vi "AssertError.vi"(8 "error in (no error)":errorcluster, 11 "Expected Error":T1=402902 items=["[5120] Invalid ID"=402902, "[5110] Failed to Init"=402900, "[5111] Unknown Error"=402901, "[5130] Save - Bad File Extension"=402903, "[5131] Save - General Error"=402904, "[5140] Unsupported (Polar)"=402905, "[5141] Unsupported (Logscale)"=402906, "[5142] Coordinates Not Regular"=402907]) -> (0 "error out":errorcluster)   [LabVIEW 2013]
uses:
  ErrorCodes.ctl
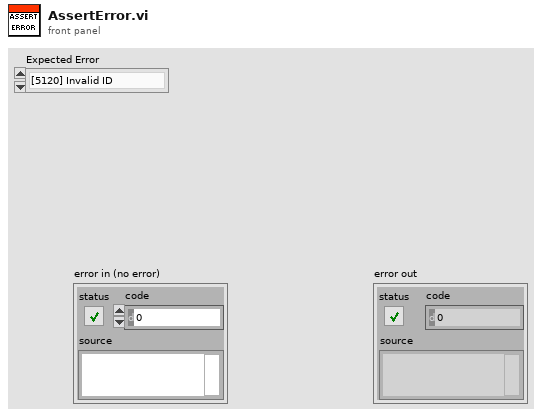
[diagram p1: front panel]
types:
  T1 = typedef "ErrorCodes.ctl" = u32
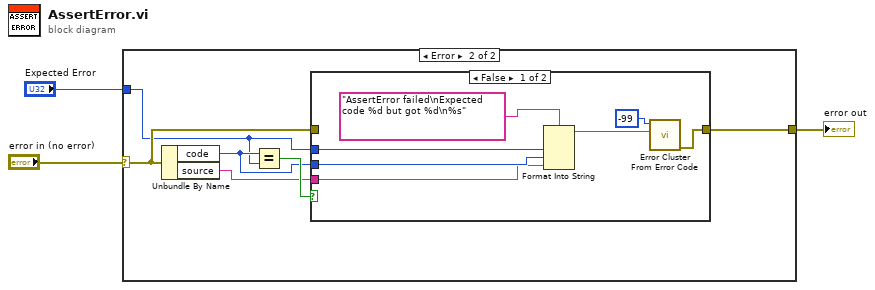
[diagram p0: block diagram]
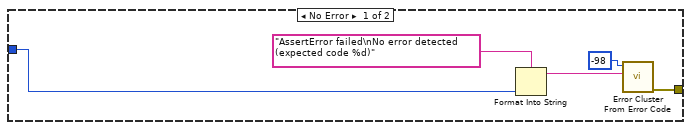
[diagram p2: hidden frame]
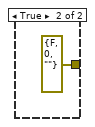
[diagram p3: hidden frame]
diagram:
  n1 = case shown="Error" "error in (no error)" {
    selector: "error in (no error)" -> [_ w13]
    tunnel: [w4 w12] -> w2
    tunnel: "Expected Error" -> [w7 w9]
    frame No Error {
      n2 = Format Into String(format string="AssertError failed\nNo error detected (expected code %d)", w7) -> (resulting string=w6:string)  [unwired: 2 in, 1 out]
      n3 = call <vilib>:"Error Cluster From Error Code.vi"("error message (\"\")"=w6, "error code (0)"=-98) -> ("error out"=w4:errorcluster)  [unwired: 7 in]
    }
    frame Error {
      n4 = Unbundle By Name(w13) -> ("code"=w11:i32, "source"=w10:string)
      n5 = Equal?(x=w11, y=w9) -> (x = y?=w14:bool)
      n6 = case shown="False" w14 {
        tunnel: w13 -> [_ _]
        tunnel: [w15 errorcluster {"status"=FALSE, "code"=0, "source"=""} ("error out")] -> w12
        tunnel: w9 -> [w20 _]
        tunnel: w11 -> [w19 _]
        tunnel: w10 -> [w18 _]
        frame False {
          n7 = Format Into String(format string="AssertError failed\nExpected code %d but got %d\n%s", w20, w19, w18) -> (resulting string=w16:string)  [unwired: 2 in, 1 out]
          n8 = call <vilib>:"Error Cluster From Error Code.vi"("error message (\"\")"=w16, "error code (0)"=-99) -> ("error out"=w15:errorcluster)  [unwired: 7 in]
        }
        frame True {
        }
      }
    }
  }
  "error out" <- w2
